vi "Pre Launch Init.vi"(11 "CoolAppProcess in":refnum<class "CoolAppProcess.lvclass">) -> (0 "error out":errorcluster, 3 "CoolAppProcess out":refnum<class "CoolAppProcess.lvclass">)   [LabVIEW 2020, in "LAF2024Q2.lvlib" / "CoolAppProcess.lvclass"]
doc: "(<B>Filename</B>: Actor Framework.lvlib:Actor.lvclass:Pre Launch Init.vi)\n\nDefines behavior that occurs after the Launch Nested Actor method is invoked but before the actor's Actor Core method begins running.\n\nBy default, this method does nothing. A descendant class may override it to define behavior."
uses:
  CoolAppProcess.lvclass
  Process State.ctl
  LAF2024Q2.lvlib
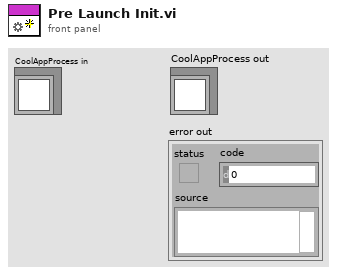
[diagram p1: front panel]
types:
  T1 = typedef "LAF2024Q2.lvlib/Process State.ctl" = enum16{"Idle", "Initializing", "Starting", "Running", "Stopping", "Stopped"}
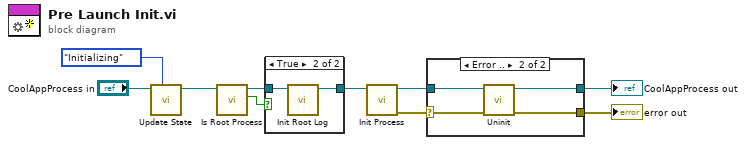
[diagram p0: block diagram]
diagram:
  n1 = call "Update State.vi"("Process State"=Process_State."Initializing", "CoolAppProcess in"="CoolAppProcess in") -> ("CoolAppProcess out"=w2:refnum<class "CoolAppProcess.lvclass">)  [unwired: 9 in]
  n2 = call "Is Root Process.vi"("CoolAppProcess in"=w2) -> ("Root Process"=w5:bool, "CoolAppProcess out"=w4:refnum<class "CoolAppProcess.lvclass">)  [unwired: 8 in, 1 out]
  n3 = case shown="True" w5 {
    tunnel: w4 -> [w11 w13]
    tunnel: [w11 w12] -> w3
    frame False {
    }
    frame True {
      n4 = call "Init Root Log.vi"("CoolAppProcess in"=w13) -> ("CoolAppProcess out"=w12:refnum<class "CoolAppProcess.lvclass">)  [unwired: 9 in, 1 out]
    }
  }
  n5 = call-dynamic "Init Process.vi"("CoolAppProcess in"=w3) -> ("error out"=w9:errorcluster, "CoolAppProcess out"=w7:refnum<class "CoolAppProcess.lvclass">)  [unwired: 9 in]
  n6 = case shown="Error .." w9 {
    selector: w9 -> [w15 w18]
    tunnel: [w15 w16] -> w8
    tunnel: w7 -> [w14 w19]
    tunnel: [w14 w17] -> w6
    frame No Error {
    }
    frame Error {
      n7 = call "Uninit.vi"("error in (no error)"=w18, "CoolAppProcess in"=w19) -> ("error out"=w16:errorcluster, "CoolAppProcess out"=w17:refnum<class "CoolAppProcess.lvclass">)  [unwired: 8 in]
    }
  }
  "error out" <- w8
  "CoolAppProcess out" <- w6
